vi "BSDL_GLOBAL_to_ComboBox.vi"() -> ()   [LabVIEW 2017]
uses:
  Saldigi_protocol_library.lvlibp
panel:
  in  "zero":bool
  in  "CHAINn/tap3":string(combo)
  in  "CHAINn/tap2":string(combo)
  in  "CHAINn/tap1":string(combo)
  in  "CHAINn in":string="chain0"
  out "debug array":string[](array[string])
  in  "CHAINn/tap0":string(combo)
  # "1st Initialize CHAINn. Then run this VI and check the values in the controls"
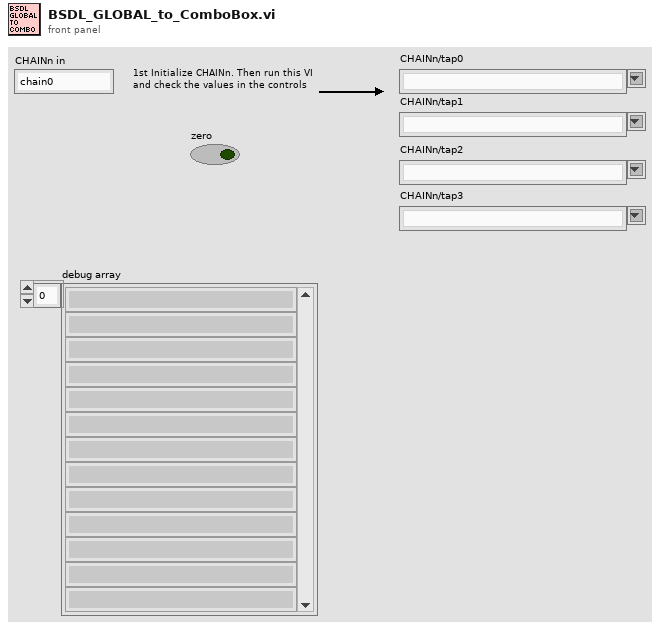
[diagram p1: front panel]
types:
  T1 = typedef "Saldigi_protocol_library.lvlibp/BSCAN_TARGET_typedef.ctl" = cluster{"BOUNDARY_REGISTER":string[][], "INSTRUCTION_OPCODE":string[][], "IDCODE_REGISTER MSB first":string, "BOUNDARY_REGISTER":bool[], "TARGET alias":string, "TARGET INSTRUCTION_REGISTER value":T2, "BOUNDARY_REGISTER last read":bool[]}
  T2 = typedef "Saldigi_protocol_library.lvlibp/BSCAN_INSTRUCTION_OPCODE_typedef.ctl" = enum16{"BYPASS", "EXTEST", "PRELOAD", "SAMPLE", "CLAMP", "HIGHZ", "INTEST", "RUNBIST", "USERCODE", "IDCODE"}
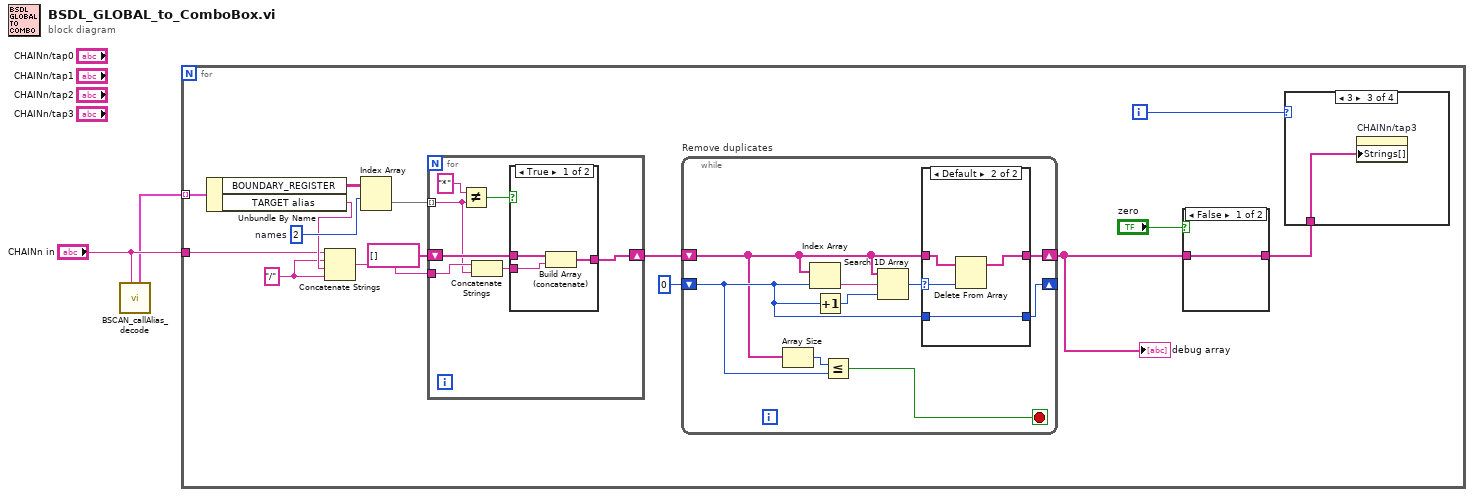
[diagram p0: block diagram]
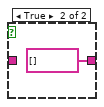
[diagram p2: hidden frame]
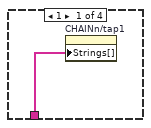
[diagram p3: hidden frame]
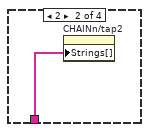
[diagram p4: hidden frame]
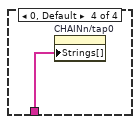
[diagram p5: hidden frame]
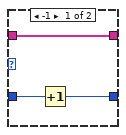
[diagram p7: hidden frame]
diagram:
  n1 = call "BSCAN_callAlias_decode.vi"("CHAINn/TARGETn/PORTn in"="CHAINn in") -> ("BSCAN CHAINn TARGET typedef array out"=w1:T1[])  [unwired: 6 in, 4 out]
  n2 = for {
    tunnel: "CHAINn in" -> [w9]
    tunnel: w1 -> [w7] mode=indexing
    i -> [w6]
    w8 = "/" ("element")
    w16 = 2  # names
    n3 = Unbundle By Name(w7) -> ("BOUNDARY_REGISTER"=w17:string[][], "TARGET alias"=w11:string)
    n4 = Concatenate Strings(w9, w8, w11, w8) -> (w10:string)
    n5 = Index Array(array=w17, index (row)=w16) -> (element=w15:string[])  [unwired: 1 in]
    n6 = for {
      tunnel: w15 -> [w25] mode=indexing
      shift-right: [w27] -> w13
      shift-left: string[] [] -> [w28]
      tunnel: w10 -> [w26]
      n7 = Not Equal?(x="*" ("y"), y=w25) -> (x != y?=w30:bool)
      n8 = Concatenate Strings(w26, w25) -> (w24:string)
      n9 = case shown="True" w30 {
        tunnel: w28 -> [w33 w34]
        tunnel: [w32 w34] -> w27
        tunnel: w24 -> [w31 _]
        frame True {
          n10 = Build Array (concatenate)(w33, w31) -> (w32:string[])
        }
        frame False {
        }
      }
    }
    n11 = while "Remove duplicates" {
      shift-right: [w40] -> _
      shift-left: 0 ("index") -> [w38]
      shift-right: [w41] -> w3
      shift-left: w13 -> [w35]
      stop <- w37 stop-if-true
      n12 = Array Size(array=w35) -> (size(s)=w39:i32)
      n13 = Index Array(array=w35, index=w38) -> (element=w43:string)
      n14 = Increment(x=w38) -> (x+1=w36:i32)
      n15 = Less Or Equal?(x=w39, y=w38) -> (x <= y?=w37:bool)
      n16 = Search 1D Array(1D array=w35, element=w43, start index (0)=w36) -> (index of element=w42:i32)
      n17 = case shown="Default" w42 {
        selector: w42 -> [_ w49]
        tunnel: w35 -> [w46 w50]
        tunnel: [w46 w48] -> w41
        tunnel: [w44 w47] -> w40
        tunnel: w38 -> [w45 w47]
        frame -1 {
          n18 = Increment(x=w45) -> (x+1=w44:i32)
        }
        frame Default {
          n19 = Delete From Array(array=w50, index=w49) -> (array with subset deleted=w48:string[])  [unwired: 1 in, 1 out]
        }
      }
    }
    "debug array" <- w3
    n20 = case shown="False" "zero" {
      tunnel: [w18 string[] []] -> w4
      tunnel: w3 -> [w18 _]
      frame False {
      }
      frame True {
      }
    }
    n21 = case shown="3" w6 {
      tunnel: w4 -> [w20 w21 w22 w23]
      frame 1 {
        n22 = property on="CHAINn/tap1" class="CmbBox"("Strings[]"=w20) -> ()  [unwired: 2 in, 2 out]
      }
      frame 2 {
        n23 = property on="CHAINn/tap2" class="CmbBox"("Strings[]"=w21) -> ()  [unwired: 2 in, 2 out]
      }
      frame 3 {
        n24 = property on="CHAINn/tap3" class="CmbBox"("Strings[]"=w22) -> ()  [unwired: 2 in, 2 out]
      }
      frame 0, Default {
        n25 = property on="CHAINn/tap0" class="CmbBox"("Strings[]"=w23) -> ()  [unwired: 2 in, 2 out]
      }
    }
  }
